vi "RT_Initialize.vi"(8 "error in":errorcluster) -> (0 "error out":errorcluster, 3 "Main Data":T1)   [LabVIEW 2018]
uses:
  Data Def/RT_Main Data.ctl
  Data Def/RT_FPGA VI Reference.ctl
  Data Def/RT_Request Data.ctl
  Data Def/RT_File Method.ctl
  Data Def/RT_Normal FGV Method.ctl
  <vilib>/FPGAPlugInAG/sbRIO-9606/niLvFpga_Open_sbRIO-9606.vi
  <vilib>/rvi/interface/common/dynamic/niFpgaDynamicAddResources.vi
  <vilib>/rvi/interface/nirviOpenFPGA/nirviOpenFPGA.xnode
  Bitfile/FPGA_Main.lvbitx
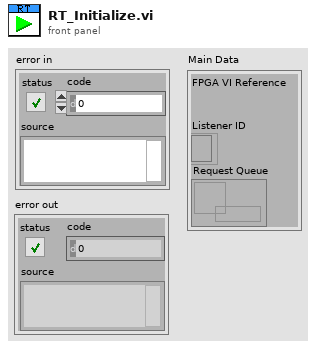
[diagram p1: front panel]
types:
  T1 = typedef "RT_Main Data.ctl" = cluster{"FPGA VI Reference":T2, "Listener ID":refnum<k5>, "Request Queue":refnum<queue>}
  T2 = typedef "RT_FPGA VI Reference.ctl" = refnum<k20>
  T3 = typedef "RT_Normal FGV Method.ctl" = enum16{"Get", "Put"}
  T4 = typedef "RT_File Method.ctl" = enum16{"Get", "Put", "Load", "Save"}
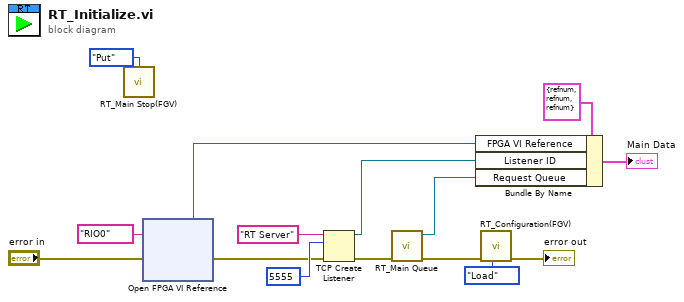
[diagram p0: block diagram]
diagram:
  n1 = call "RT_Main Stop(FGV).vi"("Normal FGV Method"=RT_Normal_FGV_Method."Put") -> ()  [unwired: 3 in, 1 out]
  n2 = xnode "Open FPGA VI Reference"("error in"="error in", "resource name"=tag "RIO0") -> ("FPGA VI Reference Out"=w5:refnum<k20>, "error out"=w6:errorcluster)
  n3 = TCP Create Listener(8:w6, 10:u16 5555 ("port"), 11:"RT Server" ("service name")) -> (0:w9:errorcluster, 3:w10:refnum<k5>)  [unwired: 2 in, 1 out]
  n4 = call "RT_Main Queue.vi"("error in"=w9) -> ("error out"=w4:errorcluster, "Request Queue"=w8:refnum<queue>)  [unwired: 9 in]
  n5 = Bundle By Name(cluster=T1 {"FPGA VI Reference"=refnum, "Listener ID"=refnum, "Request Queue"=refnum} ("Main Data"), "FPGA VI Reference"=w5, "Listener ID"=w10, "Request Queue"=w8) -> (→"Main Data":T1)
  n6 = call "RT_Configuration(FGV).vi"("File Method"=RT_File_Method."Load", "error in"=w4) -> ("error out"=→"error out":errorcluster)  [unwired: 8 in, 1 out]
